vi "Index Array Elements - double.vi"(4 "indices (none)":i32[](array[numeric])=[3, -1, 4], 7 "1D Array":dbl[](array[numeric])=[0.0, 1.0, 2.0, 3.0, 4.0]) -> (0 "output array":dbl[](array[numeric]))   [LabVIEW 2020]
doc: "Returns the elements of a 1-dimension array at indices. This is a list-based version of the built-in \"Index Array\"."
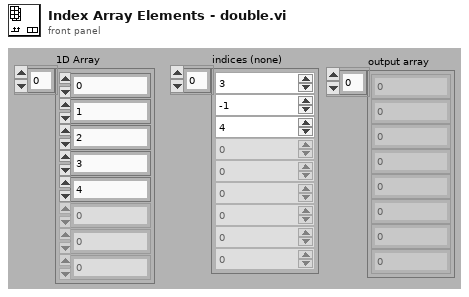
[diagram p1: front panel]
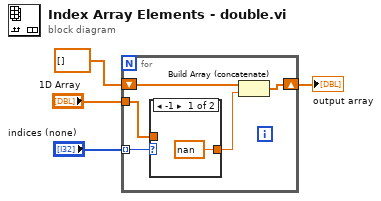
[diagram p0: block diagram]
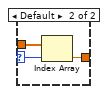
[diagram p2: hidden frame]
diagram:
  n1 = for {
    shift-right: [w6] -> w3
    shift-left: dbl[] [] ("indices (none)") -> [w8]
    tunnel: "indices (none)" -> [w5] mode=indexing
    tunnel: "1D Array" -> [w9]
    n2 = case shown="-1" w5 {
      selector: w5 -> [_ w11]
      tunnel: w9 -> [_ w13]
      tunnel: [nan ("Numeric") w12] -> w7
      frame -1 {
      }
      frame Default {
        n3 = Index Array(array=w13, index=w11) -> (element=w12:dbl)
      }
    }
    n4 = Build Array (concatenate)(w8, w7) -> (w6:dbl[])
  }
  "output array" <- w3
